vi "Read PFX Certificate.vi"(8 "error in (no error)":errorcluster, 11 "dotNET SSL Socket in":refnum<class "dotNET SSL Server.lvclass">) -> (0 "error out":errorcluster, 2 "PFX Certificate":path, 3 "dotNET SSL Socket out":refnum<class "dotNET SSL Server.lvclass">)   [LabVIEW 2013, in "dotNET SSL Socket.lvlib" / "dotNET SSL Server.lvclass"]
uses:
  dotNET SSL Server.lvclass
  dotNET SSL Server.lvclass/dotNET SSL Server.ctl
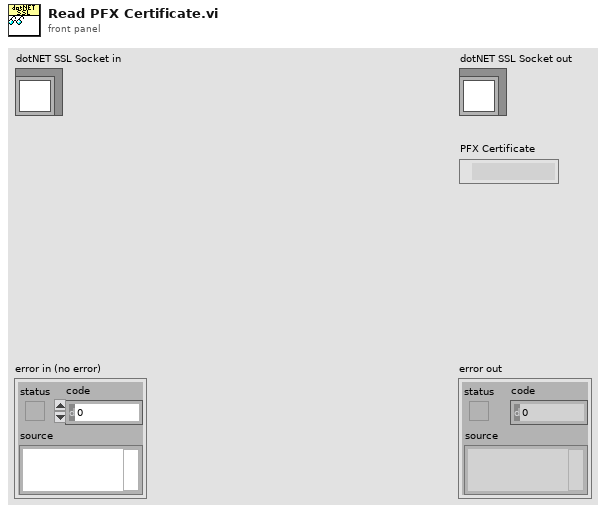
[diagram p1: front panel]
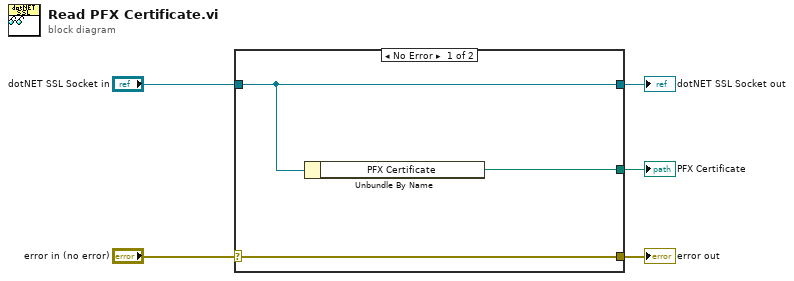
[diagram p0: block diagram]
diagram:
  n1 = case shown="No Error" "error in (no error)" {
    selector: "error in (no error)" -> [w8 w9]
    tunnel: [w8 w9] -> w4
    tunnel: [w7 w10] -> w2
    tunnel: "dotNET SSL Socket in" -> [w7 w10]
    tunnel: [w6 _] -> w1
    frame No Error {
      n2 = Unbundle By Name(w7) -> ("PFX Certificate"=w6:path)
    }
    frame Error {
    }
  }
  "error out" <- w4
  "dotNET SSL Socket out" <- w2
  "PFX Certificate" <- w1
